vi "Add Column.vi"(9 "?":string, 11 "Series in":refnum<class "Series.lvclass">) -> (3 "Series out":refnum<class "Series.lvclass">)   [LabVIEW 2018, in "InfluxDB Client.lvlib" / "Series.lvclass"]
uses:
  Series.lvclass
  Series.lvclass/Series.ctl
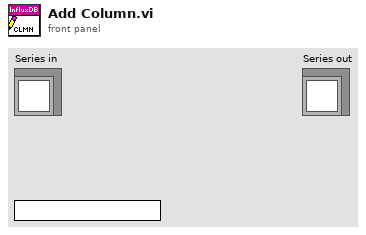
[diagram p1: front panel]
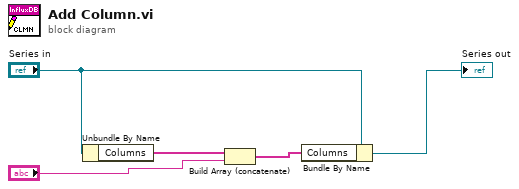
[diagram p0: block diagram]
diagram:
  n1 = Unbundle By Name("Series in") -> ("Columns"=w3:string[])
  n2 = Build Array (concatenate)(w3, "?") -> (w2:string[])
  n3 = Bundle By Name(cluster="Series in", "Columns"=w2) -> (→"Series out":refnum<class "Series.lvclass">)
